vi "Strain_Acceleration_Control.vi"() -> ()   [LabVIEW 2015]
uses:
  <vilib>/Utility/error.llb/DialogType.ctl
  <vilib>/DAQmx/read.llb/DAQmx Read (Analog Wfm 1Chan NSamp).vi
  <vilib>/Analysis/baseanly.llb/Mean (DBL).vi
  <vilib>/DAQmx/create/channels.llb/DAQmx Create Channel (AI-Voltage-Basic).vi
  <vilib>/DAQmx/configure/timing.llb/DAQmx Timing (Sample Clock).vi
  <vilib>/DAQmx/miscellaneous.llb/DAQmx Fill In Error Info.vi
  <resource>/objmgr/daqmx.rc
  <vilib>/Analysis/NI_AALPro.lvlib
  <vilib>/Analysis/NI_AALBase.lvlib
panel:
  in  "PPS address":refnum<visa-resource-name>
  in  "?":bool
  in  "?":bool
  out "Mean Voltage":dbl format="%0.3f"
  out "Accelerometer Signal [m/s^2]":cluster{dbl[], dbl[]}(graph)
  in  "Voltage for 0g":dbl
  in  "Voltage for -1g":dbl
  in  "Voltage for +1g":dbl
  in  "Set DC Voltage":dbl min=0.0 max=3.0 step=0.01
  in  "OUT on/off":bool caption="OUT"
  out "actual voltage [V]":string
  out "actual current A":string
  out "?":T1(graph)
  out "Accelerometer Signal [V]":waveform(dbl)(graph)
  in  "sample mode":i32(ring)=10178 items=["Finite Samples"=10178, "Continuous Samples"=10123, "Hardware Timed Single Point"=12522]
  in  "physical channels":tag
  in  "max voltage":dbl=5.0 format="%0.2f"
  in  "min voltage":dbl format="%0.2f"
  in  "input terminal configuration":i32(ring)=10083 items=["Default"=-1, "RSE"=10083, "NRSE"=10078, "Differential"=10106, "Pseudodifferential"=12529]
  out "OFFSET NULLING":waveform(dbl)(graph)
  out "mean unloaded":dbl format="%e"
  out "stdv unloaded":dbl format="%e"
  in  "nulling":bool
  out "?":waveform(dbl)(graph)
  out "mean loaded":dbl format="%e"
  out "stdv loaded":dbl format="%e"
  in  "Pause":bool
  out "AI.Bridge.InitialVoltage":dbl format="%_6g"
  in  "Strain physical channels":tag
  # "Motor \nand Voltage\nSource"
  # "Note: 1.19 V => 80 Hz"
  # "Strain Gauge"
  # "Accelerometer"
  # "X axis = AI4\nY axis = AI1\nZ axis = AI5\nVsup = AI0"
  # "Acceleration Calibration"
  # "Calibration: Set = mean voltage\n+1g: Accelerometer facing up\n-1g: Flip upside down\n 0g: Flip sideways"
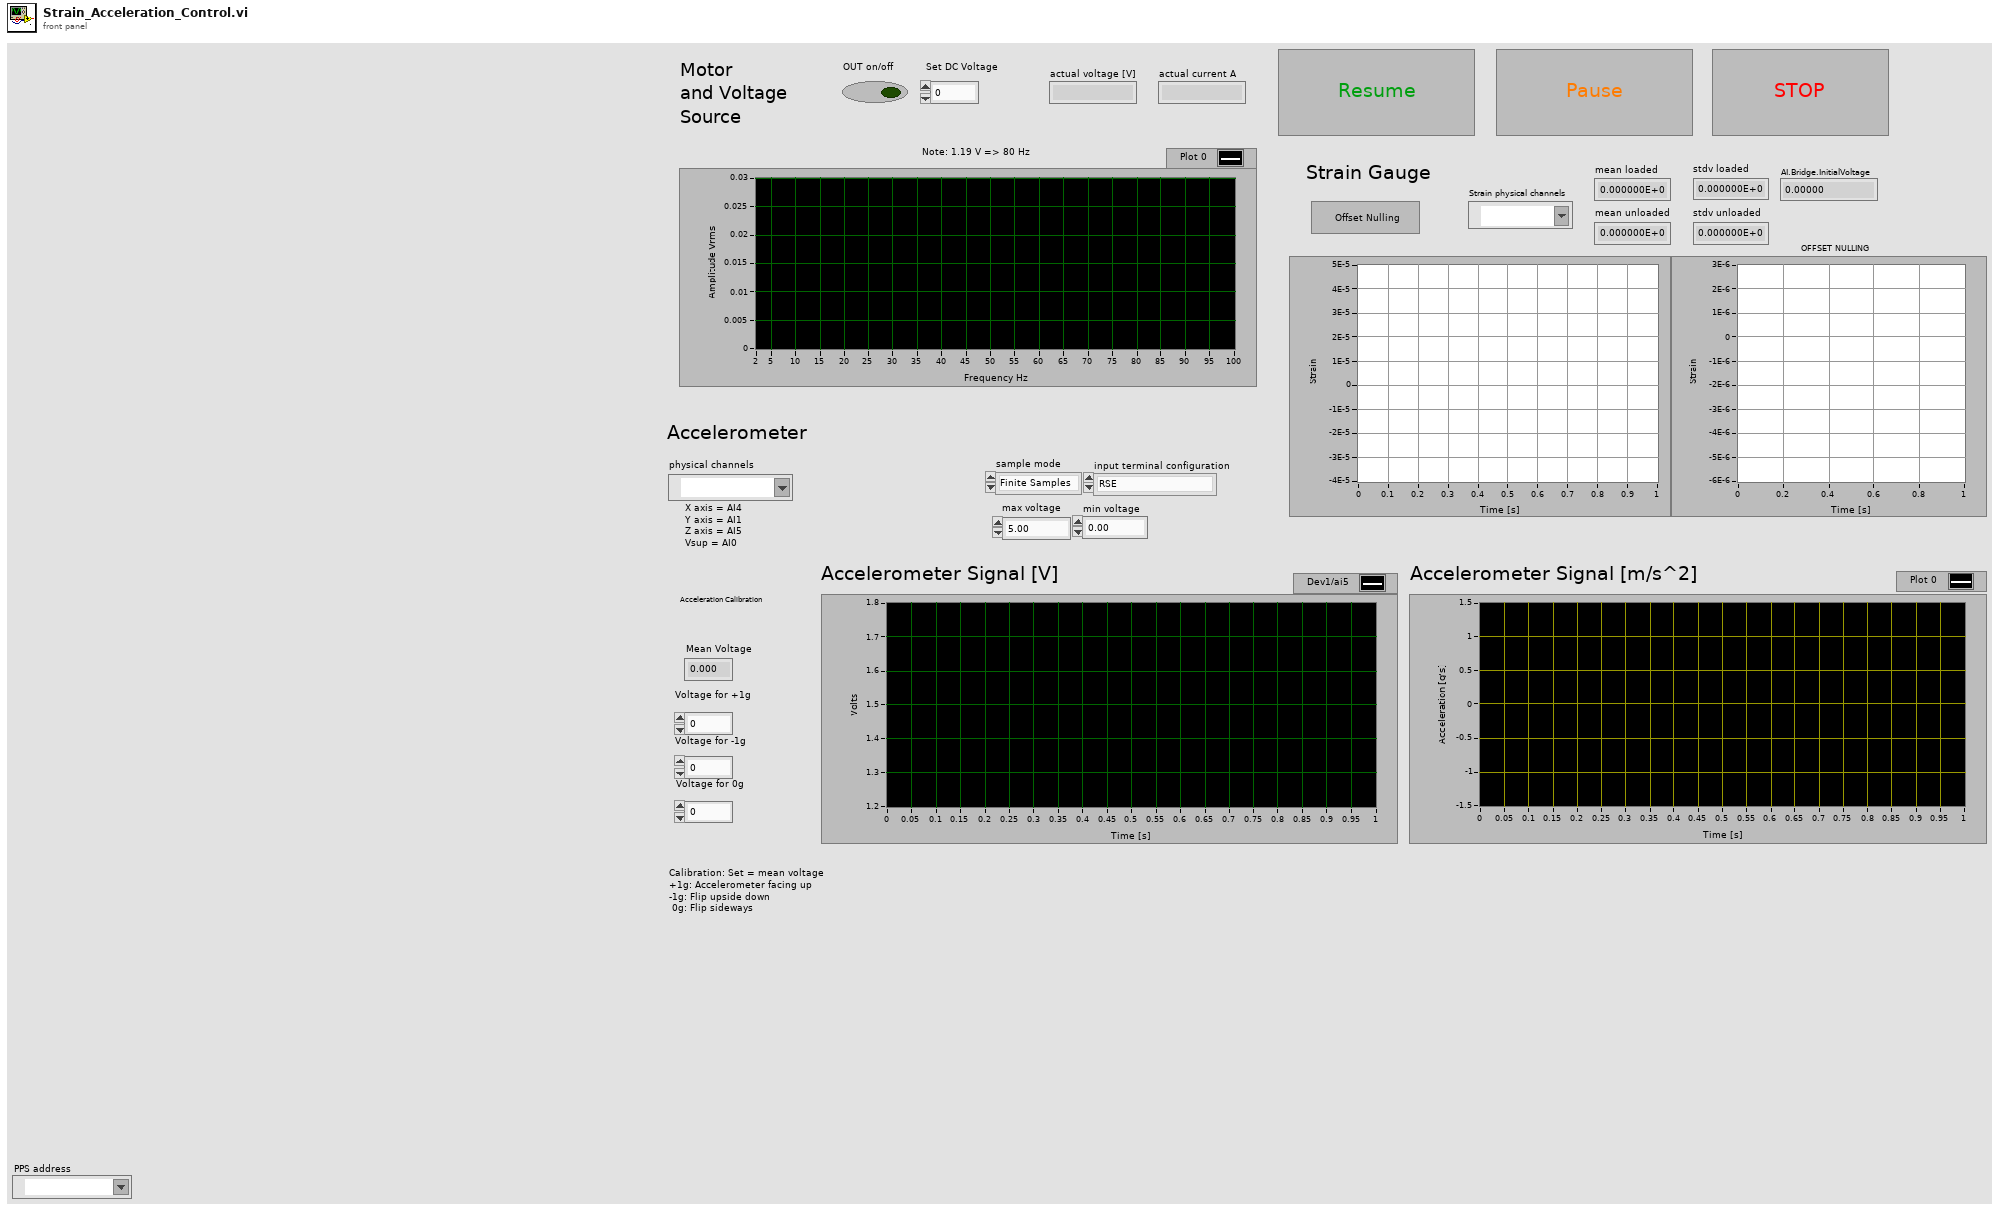
[diagram p1: front panel]
types:
  T1 = cluster{"df":dbl, "df":dbl, "Amp Spectrum Mag (Vrms)":dbl[]}
  T2 = typedef "DialogType.ctl" = u16
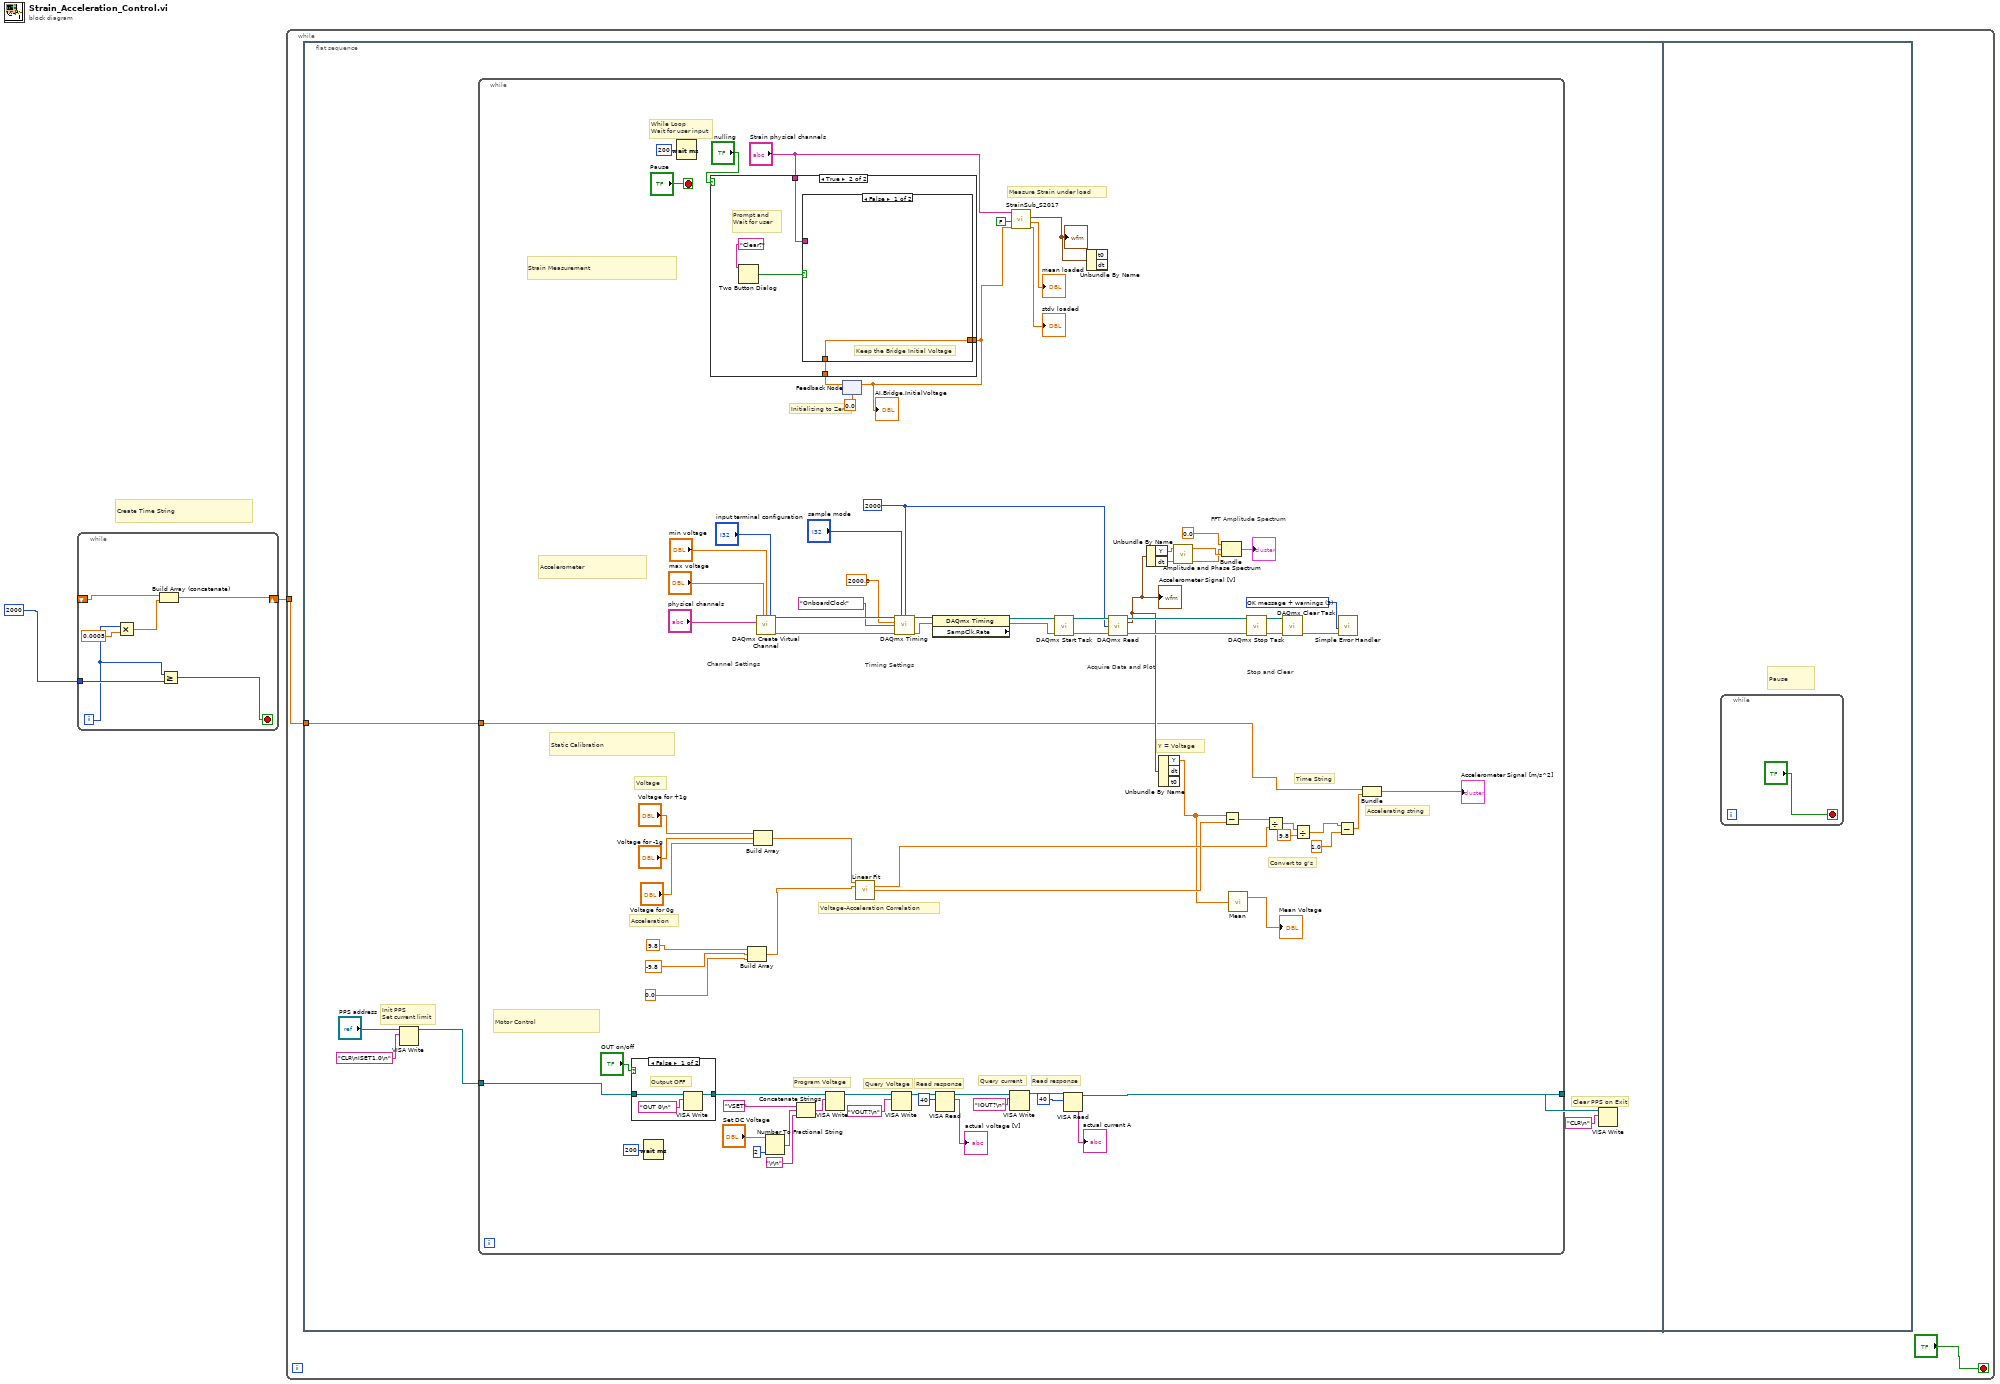
[diagram p0: block diagram]
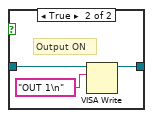
[diagram p2: hidden frame]
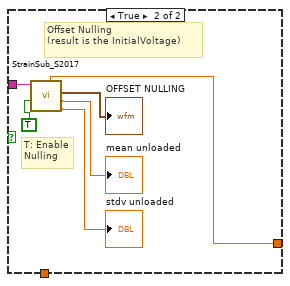
[diagram p4: hidden frame]
diagram:
  # "Create Time String"
  n1 = while {
    shift-right: [w4] -> w1
    shift-left: _ -> [w5]
    tunnel: 2000 ("dimension size") -> [w8]
    i -> [w6]
    stop <- w7 stop-if-true
    n2 = Multiply(x=w6, y=0.0005) -> (x*y=w3:dbl)
    n3 = Build Array (concatenate)(w5, w3) -> (w4:dbl[])
    n4 = Greater Or Equal?(x=w6, y=w8) -> (x >= y?=w7:bool)
  }
  n5 = while {
    tunnel: w1 -> [w11]
    stop <- "?" stop-if-true
    n6 = flat-sequence {
      tunnel: w11 -> [w15]
      frame #0 {
        # "Init PPS\nSet current limit"
        # "Clear PPS on Exit"
        n7 = VISA Write(VISA resource name="PPS address", write buffer="CLR\nISET1.0\n") -> (VISA resource name out=w12:refnum<visa-resource-name>)  [unwired: 1 in, 2 out]
        n8 = while {
          tunnel: w12 -> [w65]
          tunnel: [w64] -> w16
          tunnel: w15 -> [w21]
          stop <- "Pause" stop-if-true
          w19 = 2000 ("samples per channel")
          w66 = T2 3 items=["no dialog", "OK message", "continue or stop message", "OK message + warnings", "continue/stop + warnings"] ("type of dialog (OK msg:1)")
          # "Convert to g's"
          # "Voltage-Acceleration Correlation"
          # "Accelerating string"
          # "Time String"
          # "Y = Voltage"
          # "Stop and Clear"
          # "Acceleration"
          # "Voltage"
          # "Static Calibration"
          # "Measure Strain under load"
          # "Motor Control"
          # "Program Voltage"
          # "Read response"
          # "Query current"
          # "Read response"
          # "Query Voltage"
          # "Accelerometer"
          # "Strain Measurement"
          # "FFT Amplitude Spectrum"
          # "Acquire Data and Plot"
          # "Timing Settings"
          # "Channel Settings"
          # "While Loop\nWait for user input"
          # "Initializing to Zero"
          n9 = case shown="False" "OUT on/off" {
            tunnel: [w100 w103] -> w63
            tunnel: w65 -> [w99 w102]
            frame False {
              # "Output OFF"
              n10 = VISA Write(VISA resource name=w99, write buffer="OUT 0\n") -> (VISA resource name out=w100:refnum<visa-resource-name>)  [unwired: 1 in, 2 out]
            }
            frame True {
              # "Output ON"
              n11 = VISA Write(VISA resource name=w102, write buffer="OUT 1\n") -> (VISA resource name out=w103:refnum<visa-resource-name>)  [unwired: 1 in, 2 out]
            }
          }
          n12 = Wait (ms)(milliseconds to wait=u32 200) -> ()  [unwired: 1 out]
          n13 = Wait (ms)(milliseconds to wait=u32 200) -> ()  [unwired: 1 out]
          n14 = Build Array(9.8, -9.8, 0.0) -> (w33:dbl[])
          n15 = Build Array("Voltage for +1g", "Voltage for -1g", "Voltage for 0g") -> (w37:dbl[])
          n16 = call-poly <vilib>:"DAQmx Create Virtual Channel.vi"("maximum value"="max voltage", "minimum value"="min voltage", "input terminal configuration"="input terminal configuration", "physical channels"="physical channels") -> ("task out"=w88:refnum<k21>, "error out"=w89:errorcluster)  [unwired: 10 in]
          n17 = Number To Fractional String(number="Set DC Voltage", precision (6)=i16 2) -> (F-format string=w58:string)  [unwired: 2 in]
          n18 = Concatenate Strings("VSET" ("write buffer"), w58, "\r\n") -> (w61:string)
          n19 = VISA Write(VISA resource name=w63, write buffer=w61) -> (VISA resource name out=w47:refnum<visa-resource-name>)  [unwired: 1 in, 2 out]
          n20 = feedback #1(0.0 ("x")) -> (w94:dbl)
          n21 = case shown="True" "nulling" {
            tunnel: "Strain physical channels" -> [_ w110]
            tunnel: [w105 w106] -> w93
            tunnel: w94 -> [w105 w109]
            frame False {
              # "Keep the Bridge Initial Voltage"
            }
            frame True {
              # "Prompt and\nWait for user"
              n22 = Two Button Dialog(message="Clear?") -> (T button?=w108:bool)  [unwired: 2 in]
              n23 = case shown="False" w108 {
                tunnel: w110 -> [_ w117]
                tunnel: w109 -> [w111 _]
                tunnel: [w111 w112] -> w106
                frame False {
                  # "Keep the Bridge Initial Voltage"
                }
                frame True {
                  # "Offset Nulling\n(result is the InitialVoltage)"
                  # "T: Enable\nNulling"
                  n24 = call "StrainSub_S2017.vi"("physical channels"=w117, "Offset Null?"=TRUE ("Do Offset Null?")) -> ("AI.Bridge.InitialVoltage"=w112:dbl, "Waveform Graph"=→"OFFSET NULLING":waveform(dbl), "mean"=→"mean unloaded":dbl, "standard deviation"=→"stdv unloaded":dbl)  [unwired: 2 in, 1 out]
                }
              }
            }
          }
          "AI.Bridge.InitialVoltage" <- w93
          n25 = feedback-in #1(w93) -> ()
          n26 = call <vilib>:"Linear Fit.vi"("Y"=w37, "X"=w33) -> ("slope"=w30:dbl, "intercept"=w32:dbl)  [unwired: 9 in, 3 out]
          n27 = VISA Write(VISA resource name=w47, write buffer="VOUT?\n") -> (VISA resource name out=w48:refnum<visa-resource-name>)  [unwired: 1 in, 2 out]
          n28 = call-poly <vilib>:"DAQmx Timing.vi"("task/channels in"=w88, "sample mode"="sample mode", "samples per channel"=w19, "rate"=2000.0, "source"=tag "OnboardClock" ("clock source"), "error in"=w89) -> ("task out"=w91:refnum<k21>, "error out"=w90:errorcluster)  [unwired: 8 in]
          n29 = property class="DAQmx Timing" props=["SampClk.Rate"](reference=w91, error in=w90) -> (reference out=w83:refnum<k21>, error out=w82:errorcluster)  [unwired: 1 out]
          n30 = VISA Read(VISA resource name=w48, byte count=u32 40) -> (VISA resource name out=w55:refnum<visa-resource-name>, read buffer=→"actual voltage [V]":string)  [unwired: 1 in, 2 out]
          n31 = VISA Write(VISA resource name=w55, write buffer="IOUT?\n") -> (VISA resource name out=w53:refnum<visa-resource-name>)  [unwired: 1 in, 2 out]
          n32 = call "StrainSub_S2017.vi"("physical channels"="Strain physical channels", "Offset Null?"=FALSE, "initial bridge voltage"=w93) -> ("Waveform Graph"=w41:waveform(dbl), "mean"=→"mean loaded":dbl, "standard deviation"=→"stdv loaded":dbl)  [unwired: 1 in, 2 out]
          "?" <- w41
          n33 = call <vilib>:"DAQmx Start Task.vi"("task/channels in"=w83, "error in"=w82) -> ("task out"=w87:refnum<k21>, "error out"=w86:errorcluster)  [unwired: 12 in]
          n34 = VISA Read(VISA resource name=w53, byte count=u32 40) -> (VISA resource name out=w64:refnum<visa-resource-name>, read buffer=→"actual current A":string)  [unwired: 1 in, 2 out]
          n35 = Unbundle By Name(w41) -> ()  [unwired: 2 out]
          n36 = call-poly <vilib>:"DAQmx Read.vi"("task/channels in"=w87, "number of samples per channel"=w19, "error in"=w86) -> ("task out"=w85:refnum<k21>, "data"=w23:waveform(dbl), "error out"=w84:errorcluster)  [unwired: 10 in]
          "Accelerometer Signal [V]" <- w23
          n37 = Unbundle By Name(w23) -> ("Y"=w73:dbl[], "dt"=w72:dbl)
          n38 = Unbundle By Name(w23) -> ("Y"=w20:dbl[])  [unwired: 2 out]
          n39 = call <vilib>:"Amplitude and Phase Spectrum.vi"("dt"=w72, "Signal (V)"=w73) -> ("df"=w80:dbl, "Amp Spectrum Mag (Vrms)"=w81:dbl[])  [unwired: 1 in, 1 out]
          n40 = Bundle("df"=0.0, "df"=w80, "Amp Spectrum Mag (Vrms)"=w81) -> (→"?":T1)  [unwired: 1 in]
          n41 = Subtract(x=w20, y=w32) -> (x-y=w31:dbl[])
          n42 = call-poly <vilib>:"Mean.vi"("X"=w20) -> ("mean"=→"Mean Voltage":dbl)  [unwired: 1 out]
          n43 = call <vilib>:"DAQmx Stop Task.vi"("task/channels in"=w85, "error in"=w84) -> ("task out"=w67:refnum<k21>, "error out"=w68:errorcluster)  [unwired: 12 in]
          n44 = Divide(x=w31, y=w30) -> (x/y=w28:dbl[])
          n45 = call <vilib>:"DAQmx Clear Task.vi"("task in"=w67, "error in"=w68) -> ("error out"=w69:errorcluster)  [unwired: 13 in]
          n46 = Divide(x=w28, y=9.8) -> (x/y=w27:dbl[])
          n47 = Subtract(x=w27, y=1.0) -> (x-y=w22:dbl[])
          n48 = call <vilib>:"Simple Error Handler.vi"("type of dialog (OK msg:1)"=w66, "error in (no error)"=w69) -> ()  [unwired: 3 in, 5 out]
          n49 = Bundle(w21, w22) -> (→"Accelerometer Signal [m/s^2]":cluster{dbl[], dbl[]})  [unwired: 1 in]
        }
        n50 = VISA Write(VISA resource name=w16, write buffer="CLR\n") -> ()  [unwired: 1 in, 3 out]
      }
      frame #1 {
        # "Pause"
        n51 = while {
          stop <- "?" stop-if-true
        }
      }
    }
  }
